vi "rotate 2D array V5.vi"(9 "rotate y":i32=1, 10 "rotate x":i32, 11 "array in":cdb[][](array[numeric])=[[0.0+0.0i, 1.0+0.0i, 2.0+0.0i, 3.0+0.0i], [4.0+0.0i, 0.0+0.0i, 0.0+0.0i, 0.0+0.0i], [8.0+0.0i, 0.0+0.0i, 0.0+0.0i, 0.0+0.0i], [13.0+0.0i, 0.0+0.0i, 99.0+0.0i, 0.0+0.0i]]) -> (3 "array out":cdb[][](array[numeric])=[[13.0+0.0i, 0.0+0.0i, 99.0+0.0i, 0.0+0.0i], [0.0+0.0i, 1.0+0.0i, 2.0+0.0i, 3.0+0.0i], [4.0+0.0i, 0.0+0.0i, 0.0+0.0i, 0.0+0.0i], [8.0+0.0i, 0.0+0.0i, 0.0+0.0i, 0.0+0.0i]])   [LabVIEW 2010]
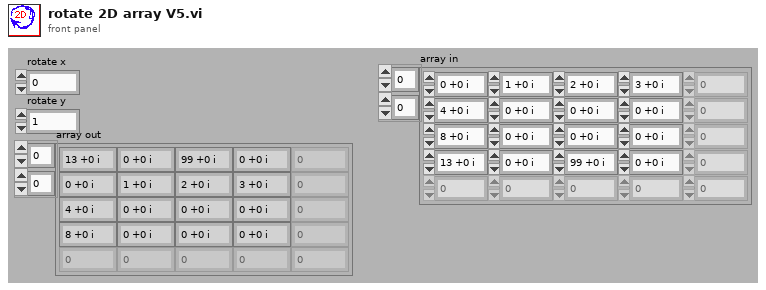
[diagram p1: front panel]
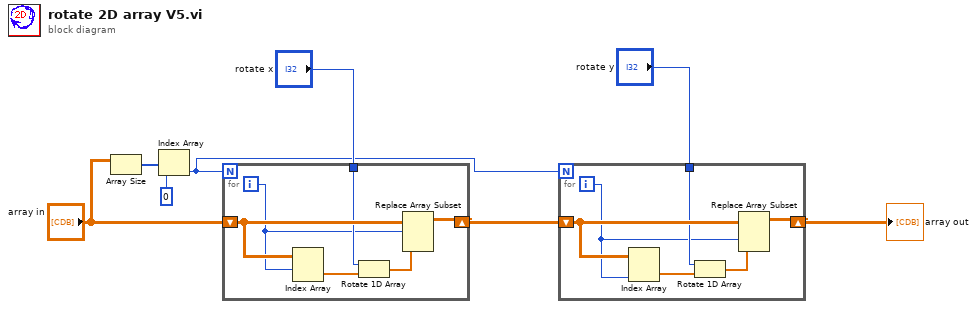
[diagram p0: block diagram]
diagram:
  n1 = Array Size(array="array in") -> (size(s)=w7:i32[])
  n2 = Index Array(array=w7, index=0) -> (element=w1:i32)
  n3 = for {
    N: w1 -> [_]
    shift-right: [w14] -> w4
    shift-left: "array in" -> [w13]
    tunnel: "rotate x" -> [w10]
    i -> [w9]
    n4 = Index Array(array=w13, index (row)=w9) -> (element=w11:cdb[])  [unwired: 1 in]
    n5 = Rotate 1D Array(1:w11, 2:w10) -> (0:w12:cdb[])
    n6 = Replace Array Subset(array=w13, new element=w12, index (row)=w9) -> (w14:cdb[][])  [unwired: 1 in]
  }
  n7 = for {
    N: w1 -> [_]
    shift-right: [w20] -> w3
    shift-left: w4 -> [w19]
    tunnel: "rotate y" -> [w16]
    i -> [w15]
    n8 = Index Array(array=w19, index (col)=w15) -> (element=w17:cdb[])  [unwired: 1 in]
    n9 = Rotate 1D Array(1:w17, 2:w16) -> (0:w18:cdb[])
    n10 = Replace Array Subset(array=w19, new element=w18, index (col)=w15) -> (w20:cdb[][])  [unwired: 1 in]
  }
  "array out" <- w3
